vi "Read Integrate Configuration.vi"(8 "error in (no error)":errorcluster, 11 "Integrate in":refnum<class "Integrate.lvclass">) -> (0 "error out":errorcluster, 2 "Configuration":T1={"Integrate"=[], "Offset duration "=0.0095, "TDMS group name"="p"} {"Offset duration" format="%#_6ps"; "Integrate"."Duration" format="%#_6ps"; "Integrate"."Start time" format="%#_6ps"}, 3 "Integrate out":refnum<class "Integrate.lvclass">)   [LabVIEW 2016, in "Integrate.lvclass"]
uses:
  Integrate.lvclass
  C:/github/LabActor/Template Module/Template Module.lvclass
  Integrator Configuration.ctl
  NHMFL_Core/Libraries/Utilities/Controls/Integrate channel.ctl
  Template Module/Template Module.lvclass/Template Module.ctl
  Template Module/Read Configuration.vi
panel:
  # "Input CH"
  # "X-Factor"
  # "Output CH"
  # "Start"
  # "Duration"
  # "Fix drift"
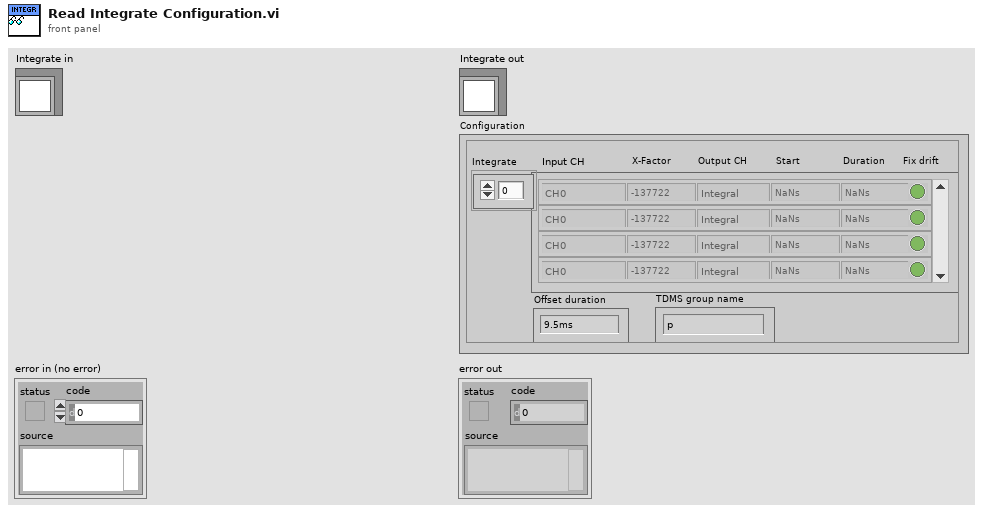
[diagram p1: front panel]
types:
  T1 = typedef "Integrator Configuration.ctl" = cluster{"Integrate":T2[], "Offset duration ":dbl, "TDMS group name":string}
  T2 = typedef "Integrate channel.ctl" = cluster{"Channel":string, "Output name":string, "Factor":dbl, "Start time":dbl, "Duration":dbl, "Fix drift":bool}
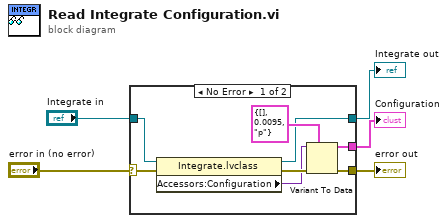
[diagram p0: block diagram]
diagram:
  n1 = case shown="No Error" "error in (no error)" {
    selector: "error in (no error)" -> [w9 w14]
    tunnel: [w10 w14] -> w4
    tunnel: [w6 w15] -> w2
    tunnel: "Integrate in" -> [w7 w15]
    tunnel: [w8 _] -> w1
    frame No Error {
      n2 = property class="Integrate.lvclass"(reference=w7, error in=w9) -> (reference out=w6:refnum<class "Integrate.lvclass">, error out=w13:errorcluster, "Accessors:Configuration"=w12:variant)
      n3 = Variant To Data(error in=w13, type=T1 {"Integrate"=[], "Offset duration "=0.0095, "TDMS group name"="p"} ("Configuration"), Variant=w12) -> (data=w8:T1, error out=w10:errorcluster)
    }
    frame Error {
    }
  }
  "error out" <- w4
  "Integrate out" <- w2
  "Configuration" <- w1
